vi "Boolean String to Boolean.vi"(7 "Boolean String (empty - FALSE)":string) -> (3 "Boolean":bool)   [LabVIEW 2011]
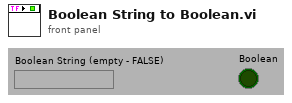
[diagram p1: front panel]
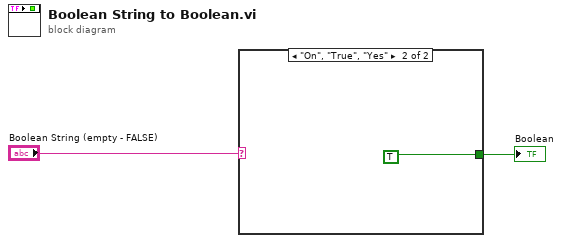
[diagram p0: block diagram]
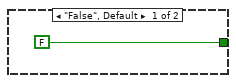
[diagram p2: hidden frame]
diagram:
  n1 = case shown="\"On\", \"True\", \"Yes\"" "Boolean String (empty - FALSE)" {
    tunnel: [FALSE TRUE] -> w1
    frame "False", Default {
    }
    frame "On", "True", "Yes" {
    }
  }
  "Boolean" <- w1
